vi "Write Output_Enable.vi"(8 "error in":errorcluster, 10 "Output_Enable":bool, 11 "IF_XX in":refnum<class "IF_XX.lvclass">) -> (0 "error out":errorcluster, 3 "IF_XX out":refnum<class "IF_XX.lvclass">)   [LabVIEW 2019, in "IF_XX.lvlib" / "IF_XX.lvclass"]
doc: "This should toggle the output enable state."
uses:
  Library/IF_XX.lvclass
  Library/IF_XX.lvclass/IF_XX.ctl
  builds/Instruments/PowerSupply.lvlibp/Library/PowerSupply.lvclass
panel:
  out "Read data":string
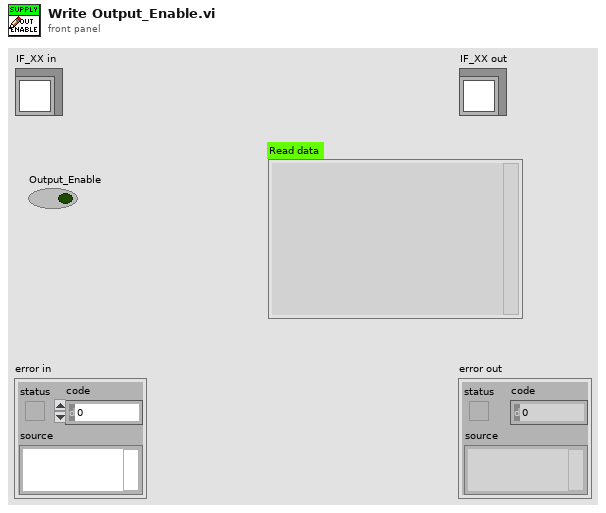
[diagram p1: front panel]
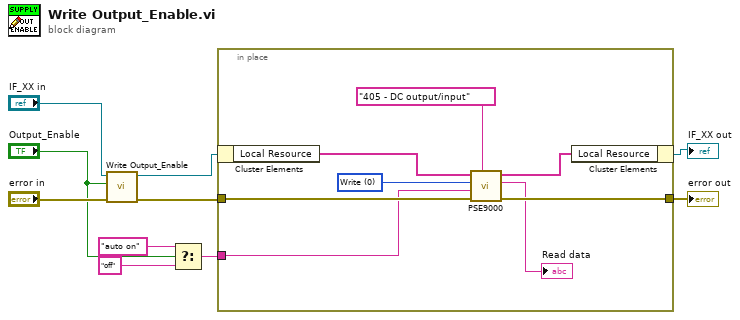
[diagram p0: block diagram]
diagram:
  n1 = call-parent "Write Output_Enable.vi"("error in"="error in", "Output_Enable"="Output_Enable", "PowerSupply in"="IF_XX in") -> ("error out"=w8:errorcluster, "PowerSupply out"=w5:refnum<class "IF_XX.lvclass">)  [unwired: 7 in]
  n2 = Select(t="auto on", s="Output_Enable", f="off") -> (s? t:f=w1:string)
  n3 = in-place {
    in-place-border: w8 -> [w18]
    in-place-border: [w17] -> w7
    in-place-border: w1 -> [w11]
    w14 = u8 0 items=["Write", "Read"] ("Access")
    n4 = in-place-cluster #1(w5) -> ("Local Resource"=w16:string[])
    n5 = call <instrlib>:"PSE9000.vi"("Command list"="405 - DC output/input", "Error in"=w18, "Value"=w11, "Access"=w14, "Device information in"=w16) -> ("Error out"=w17:errorcluster, "Read data"=→"Read data":string, "Device information out"=w15:string[])  [unwired: 1 in, 1 out]
    n6 = in-place-cluster #1("Local Resource"=w15) -> (→"IF_XX out":refnum<class "IF_XX.lvclass">)
  }
  "error out" <- w7
